vi "VI Tree - comparison.vi"   [LabVIEW 2020]
uses:
  Data Changed/Variant Changed.vi
  openg_comparison.lvlib
panel:
  # "[OpenG VI Tags] ***Do Not Remove***"
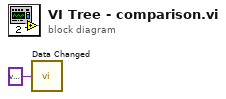
[diagram p0: block diagram]
diagram:
  n1 = call-poly "Data Changed.vi"("Variant"=variant) -> ()  [unwired: 1 out]
